vi "Record Samples (global).vi"() -> ()   [LabVIEW 2019]
panel:
  in  "Record Samples":i32
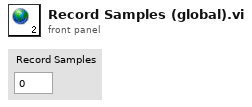
[diagram p1: front panel]
diagram:
